vi "Read Record Data.vi"(8 "Error In (no error)":errorcluster, 11 "Expenses Tracker Subcategory In":refnum<class "Expenses Tracker Subcategory.lvclass">) -> (0 "Error Out":errorcluster, 2 "Record":variant, 3 "Expenses Tracker Subcategory Out":refnum<class "Expenses Tracker Subcategory.lvclass">)   [LabVIEW 2023, in "Expenses Tracker Subcategory.lvclass"]
uses:
  Expenses Tracker Subcategory.lvclass
  Expenses Tracker Subcategory.lvclass/Expenses Tracker Subcategory.ctl
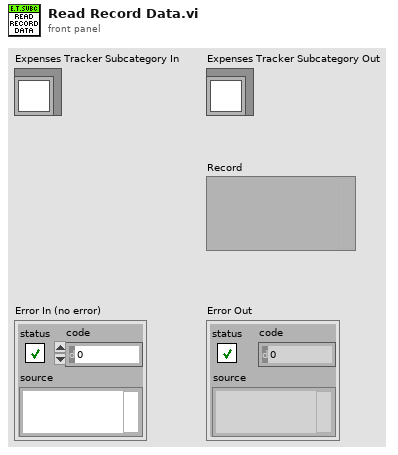
[diagram p1: front panel]
types:
  T1 = typedef "Expenses Tracker Subcategory.lvclass/Subcategory.ctl" = cluster{"ID":u32, "Name":string, "Category":u32}
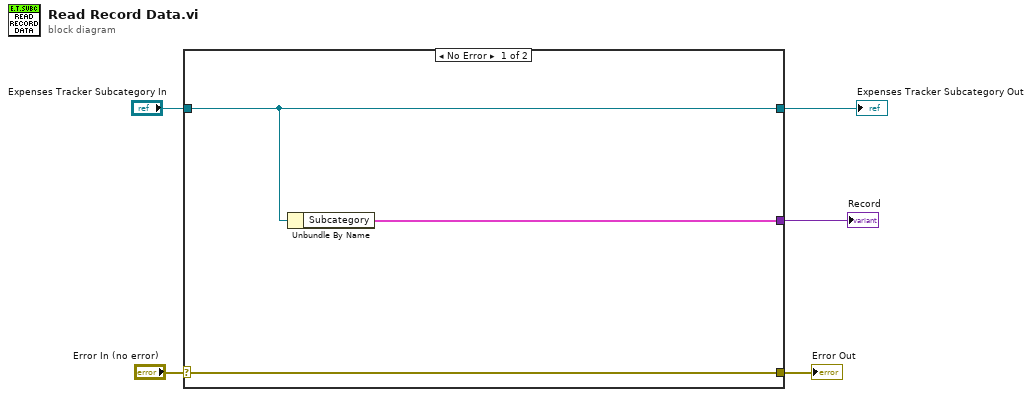
[diagram p0: block diagram]
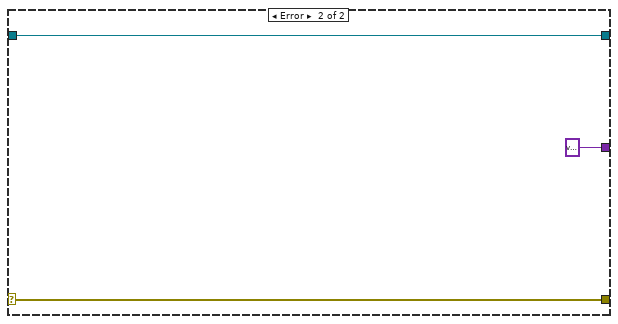
[diagram p2: hidden frame]
diagram:
  n1 = case shown="No Error" "Error In (no error)" {
    selector: "Error In (no error)" -> [w8 w11]
    tunnel: [w8 w11] -> w2
    tunnel: [w7 w10] -> w5
    tunnel: "Expenses Tracker Subcategory In" -> [w7 w10]
    tunnel: [w6 variant] -> w1
    frame No Error {
      n2 = Unbundle By Name(w7) -> ("Subcategory"=w6:T1)
    }
    frame Error {
    }
  }
  "Error Out" <- w2
  "Expenses Tracker Subcategory Out" <- w5
  "Record" <- w1
